vi "6-1.vi"() -> ()   [LabVIEW 2022 SP3, in "AoC22.lvlib"]
uses:
  AoC22.lvlib
panel:
  out "Numeric":i32
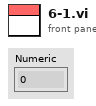
[diagram p1: front panel]
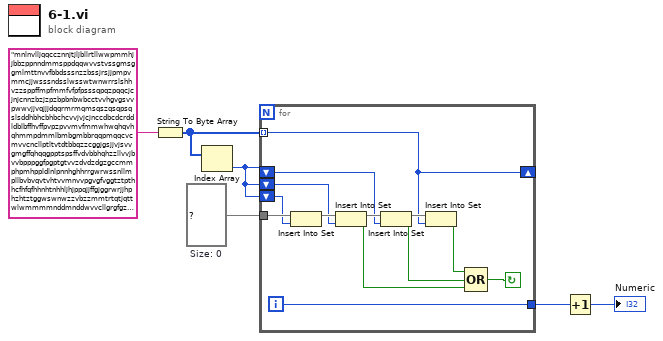
[diagram p0: block diagram]
diagram:
  w1 = set{u8} {}  # Size: 0
  n1 = String To Byte Array(string="mnlnvlljqqccznnjtjljbllrtllwwpmmhjjbbzppnndmmsppdqqwvvstvssgmsggmlmttnvvfbbdsssnzzbssjrsjjpmpvmmcjjwsssndsslwsswtwnwrrslshhvzzsppffmpfmmfvfpfpsssqpqzpqqcjcjnjcnnzbzjzpzbpbnbwbcctvvhgvgsvvpwwvjjvqjjjdqqrmrmqmsqszqsqpsqslsddhbhcbhbchcvvjvjcjnccdbcdcrddldblbffhvffpvpzpvvmvfmmwhwqhqvhqhmmpdmmlbmbgmbbrqqpmqqcvcmvvcncllptltvtdtbbqzzcggjgsjjvjsvvgmgffqhqqgpptspsffvdvbbhqhzzllvvjbvvbpppggfpgptgtvvzdvdzdgzgccmmphpmhppldlnlpnnhghhrrgwrwssnllmpllbvbvqvtvhtvvmnvvpgvgfvggtztpthhcfhfqfhhnhtnhhljhjppqjjffgjggrwrjjhphzhtztggwswnwzzvbzzmmtrtqtjqttwlwmmmmnddmnddwvvcllgrgfgzznwnsswjjhwwspsbbvzzqvzvbvcvmmtltnlnfn...") -> (unsigned byte array=w3:u8[])
  n2 = Index Array(array=w3) -> (element=w2:u8)  [unwired: 1 in]
  n3 = for {
    tunnel: w3 -> [w10] mode=indexing
    shift-right: [w10] -> _
    shift-left: w2 -> [w11]
    shift-left: w2 -> [w12]
    shift-left: w2 -> [w16]
    tunnel: [w18] -> w5
    tunnel: w1 -> [w17]
    i -> [w18]
    stop <- w19 continue-if-true
    n4 = Insert Into Set(10:w16, 11:w17) -> (3:w15:set{u8})  [unwired: 1 out]
    n5 = Insert Into Set(10:w12, 11:w15) -> (2:w9:bool, 3:w14:set{u8})
    n6 = Insert Into Set(10:w11, 11:w14) -> (2:w8:bool, 3:w13:set{u8})
    n7 = Insert Into Set(10:w10, 11:w13) -> (2:w7:bool)  [unwired: 1 out]
    n8 = Compound Arithmetic op=OR(w7, w8, w9) -> (w19:bool)
  }
  n9 = Increment(x=w5) -> (x+1=→"Numeric":i32)
